vi "Interpolation.vi"(1 "Number of Columns":i32, 2 "Lambda Interval":dbl[](array[numeric]) format="%_6g", 3 "Illuminants":string[][](array[string])) -> (0 "Interpolated":dbl[][](array[numeric]))   [LabVIEW 2014]
uses:
  <vilib>/gmath/NI_Gmath.lvlib
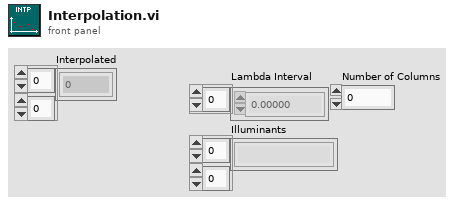
[diagram p1: front panel]
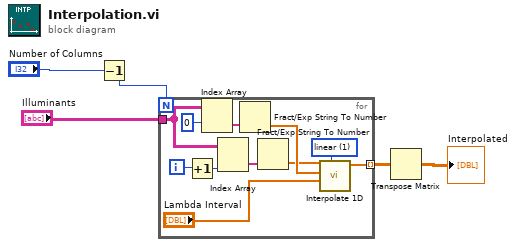
[diagram p0: block diagram]
diagram:
  n1 = Decrement(x="Number of Columns") -> (x-1=w4:i32)
  n2 = for {
    N: w4 -> [_]
    tunnel: "Illuminants" -> [w13]
    tunnel: [w10] -> w5 mode=indexing
    i -> [w9]
    w7 = 1 items=["nearest", "linear", "spline", "cubic Hermite", "Lagrange"] ("method")
    n3 = Increment(x=w9) -> (x+1=w8:i32)
    n4 = Index Array(array=w13, index (col)=0 ("disabled index (col)")) -> (element=w15:string[])  [unwired: 1 in]
    n5 = Index Array(array=w13, index (col)=w8) -> (element=w12:string[])  [unwired: 1 in]
    n6 = Fract/Exp String To Number(string=w15) -> (number=w14:dbl[])  [unwired: 3 in, 1 out]
    n7 = Fract/Exp String To Number(string=w12) -> (number=w11:dbl[])  [unwired: 3 in, 1 out]
    n8 = call <vilib>:"Interpolate 1D.vi"("method"=w7, "xi"="Lambda Interval", "X"=w14, "Y"=w11) -> ("yi"=w10:dbl[])  [unwired: 5 in, 2 out]
  }
  n9 = Transpose Matrix(1:w5) -> (0:→"Interpolated":dbl[][])
